vi "ziLoadFactory.vi"(4 "error in":errorcluster, 7 "Handle In":T1 {"Handle" format="0x%08x"; "Conn" format="0x%08x"}) -> (0 "error out":errorcluster, 3 "Handle Out":T1 {"Handle" format="0x%08x"; "Conn" format="0x%08x"})   [LabVIEW 2009, in "Zurich Instruments LabOne.lvlib"]
doc: "This resets the device to factory default. Warning: HF2 not supported"
uses:
  <instrlib>/Zurich Instruments LabOne/Zurich Instruments LabOne.lvlib
  <instrlib>/Zurich Instruments LabOne/Public/ziTypeHandle.ctl
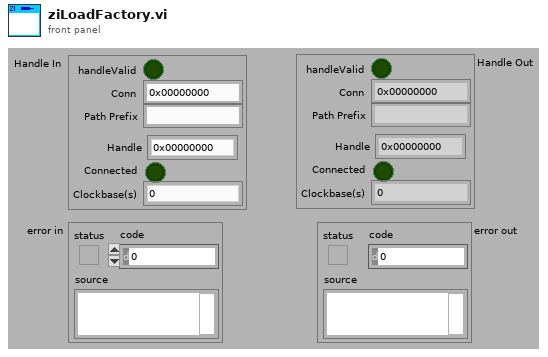
[diagram p1: front panel]
types:
  T1 = typedef "Zurich Instruments LabOne.lvlib/ziTypeHandle.ctl" = cluster{"handleValid":bool, "Conn":u64, "Path Prefix":string, "Handle":u64, "Connected":bool, "Clockbase(s)":dbl}
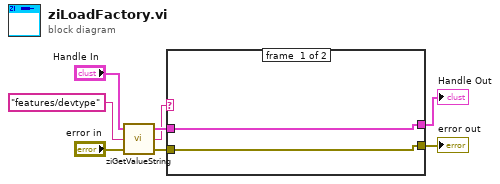
[diagram p0: block diagram]
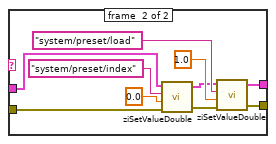
[diagram p2: hidden frame]
diagram:
  n1 = call <instrlib>:"ziGetValueString.vi"("error in"="error in", "Path"="features/devtype", "Handle In"="Handle In") -> ("error out"=w4:errorcluster, "Value"=w1:string, "Handle Out"=w2:T1)
  n2 = case shown="\"HF2LI\"" w1 {
    tunnel: [w9 w19] -> w8
    tunnel: [w10 w13] -> w7
    tunnel: w4 -> [w9 w12]
    tunnel: w2 -> [w10 w11]
    frame #0 {
    }
    frame #1 {
      n3 = call <instrlib>:"ziSetValueDouble.vi"("Error In"=w12, "Value"=0.0, "Path"="system/preset/index", "Handle In"=w11) -> ("Error Out"=w20:errorcluster, "Handle Out"=w14:T1)  [unwired: 1 in]
      n4 = call <instrlib>:"ziSetValueDouble.vi"("Error In"=w20, "Value"=1.0, "Path"="system/preset/load", "Handle In"=w14) -> ("Error Out"=w19:errorcluster, "Handle Out"=w13:T1)  [unwired: 1 in]
    }
  }
  "Handle Out" <- w7
  "error out" <- w8
